vi "Init Msg Default.vi"() -> (2 "Msg":refnum<class "Msg.lvclass">)   [LabVIEW 2025, in "_Template.lvlib" / "Templates.lvlib" / "TEMPLATE jettl Msg.lvlib"]
uses:
  TEMPLATE jettl Msg.lvlib
  TEMPLATE Msg/TEMPLATE Msg.lvlib
  jettl/jettl/Msg Input/Msg Input.lvclass
  jettl/jettl/Msg/Msg.lvclass
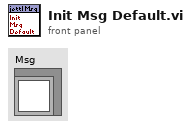
[diagram p1: front panel]
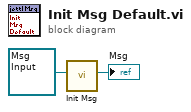
[diagram p0: block diagram]
diagram:
  n1 = call "Init Msg.vi"("Msg Input"=refnum<class "Msg Input.lvclass"> refnum) -> ("Msg"=→"Msg":refnum<class "Msg.lvclass">)  [unwired: 10 in]
